vi "Config Sequence.vi"(8 "error in (no error)":errorcluster, 11 "STEPs":T1[](array[typedef])) -> (0 "error out":errorcluster, 3 "STEPs Out":T1[](array[typedef]))   [LabVIEW 2014, in "SeqLoop.lvlib"]
doc: "Configura las Mediciones."
uses:
  SeqLoop.lvlib
  TypeDefs/STEP.ctl
  TypeDefs/LogicParsedExpression.ctl
  Mimico Display/TypeDefs/Mimic Data.ctl
  Mimico Display/TypeDefs/BG Image.ctl
  Mimico Display/TypeDefs/mObject.ctl
  <vilib>/regexp/Match Regular Expression.xnode
  Mimico Display/Mimico Display.lvlib
panel:
  in  "Ver Seq":bool
  in  "Stop Seq":bool
  in  "Delete Seq":bool
  in  "Add Seq":bool
  in  "Secuencias":i32(listbox)=-1 caption="Secuencia"
  in  "Edit Seq":bool
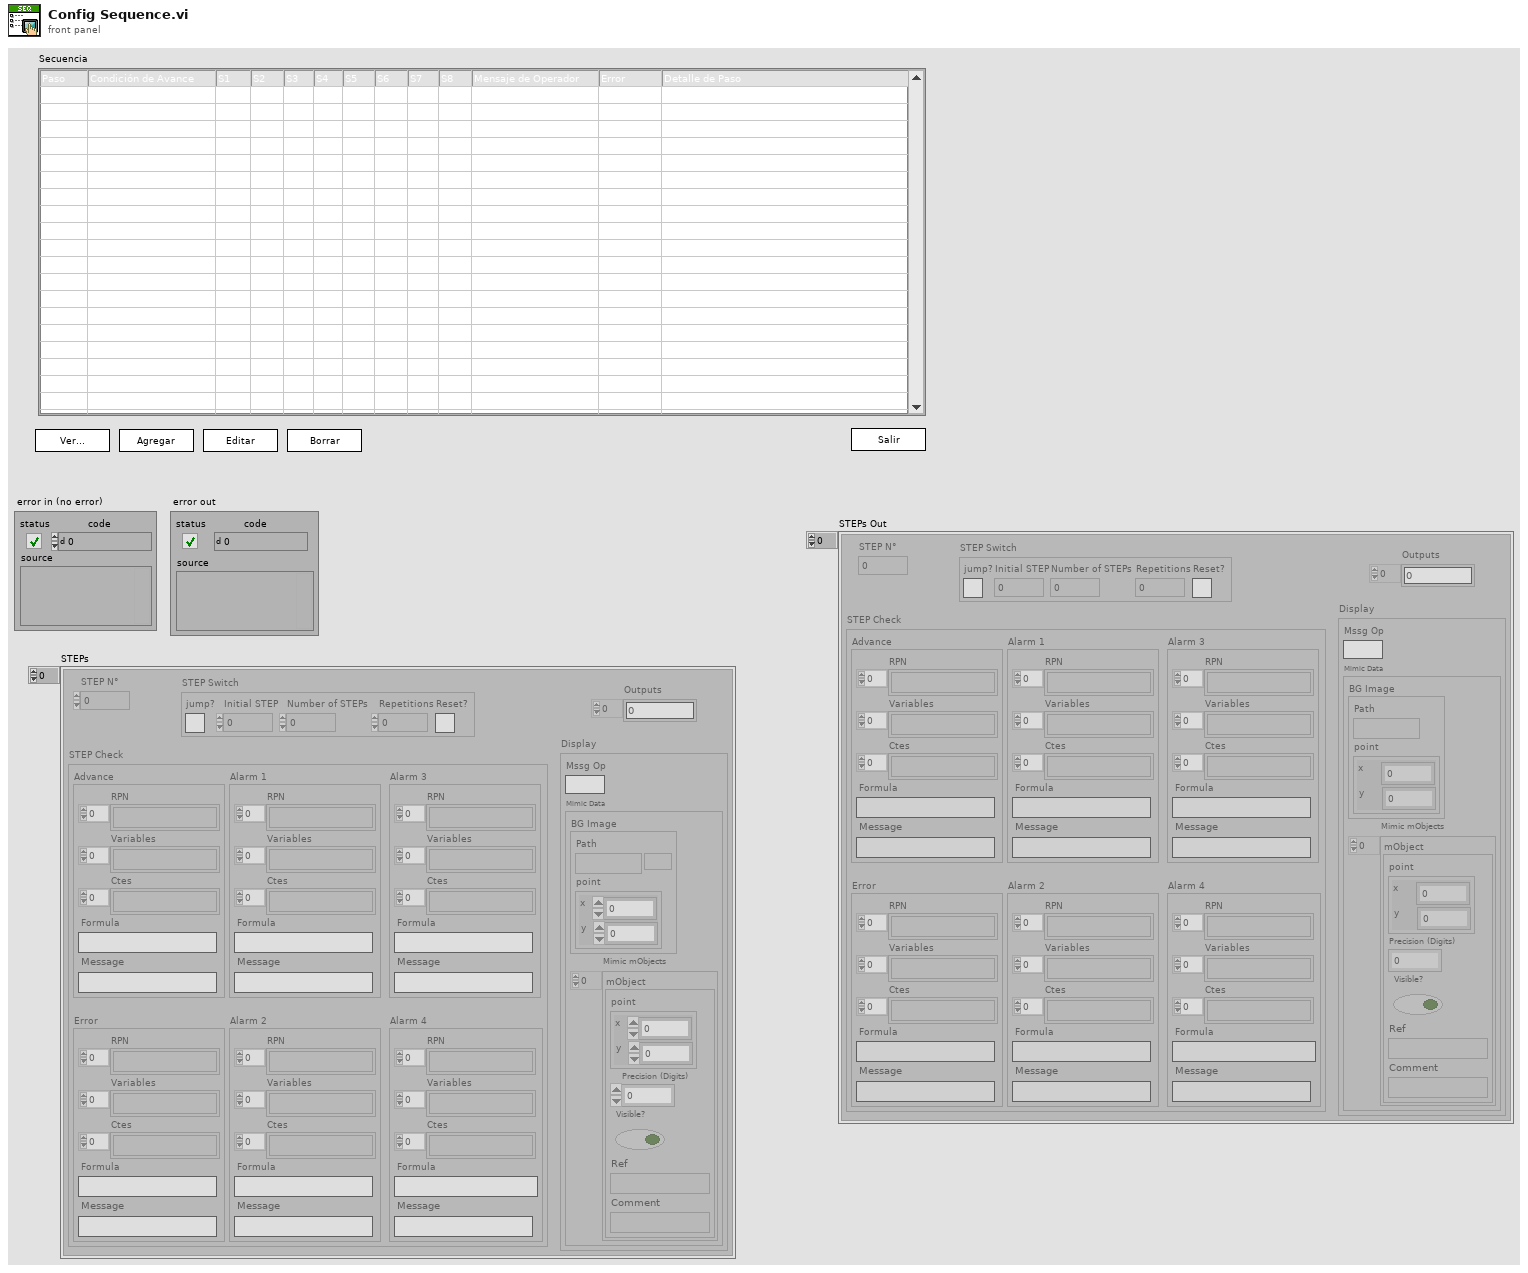
[diagram p1: front panel]
types:
  T1 = typedef "SeqLoop.lvlib/STEP.ctl" = cluster{"STEP N°":u32, "STEP Switch":cluster{"jump?":bool, "Initial STEP":u32, "Number of STEPs":u32, "Repetitions":u32, "Reset?":bool}, "Outputs":i32[], "STEP Check":cluster{"Advance":T2, "Error ":T2, "Alarm 1":T2, "Alarm 2":T2, "Alarm 3":T2, "Alarm 4":T2}, "Display":cluster{"Mssg Op":string, "Mimic Data":T3}}
  T2 = typedef "SeqLoop.lvlib/LogicParsedExpression.ctl" = cluster{"RPN ":string[], "Variables":string[], "Ctes":string[], "Formula":string, "Message":string}
  T3 = typedef "SeqLoop.lvlib/Mimico Display.lvlib/Mimic Data.ctl" = cluster{"BG Image":T4, "Mimic mObjects":T5[]}
  T4 = typedef "SeqLoop.lvlib/Mimico Display.lvlib/BG Image.ctl" = cluster{"Path":path, "point":cluster{"x":i16, "y":i16}}
  T5 = typedef "SeqLoop.lvlib/Mimico Display.lvlib/mObject.ctl" = cluster{"point":cluster{"x":i16, "y":i16}, "Precision (Digits)":i32, "Visible?":bool, "Ref":string, "Comment":string}
  T6 = enum8{"Enabled", "Disabled", "Disabled and Grayed Out"}
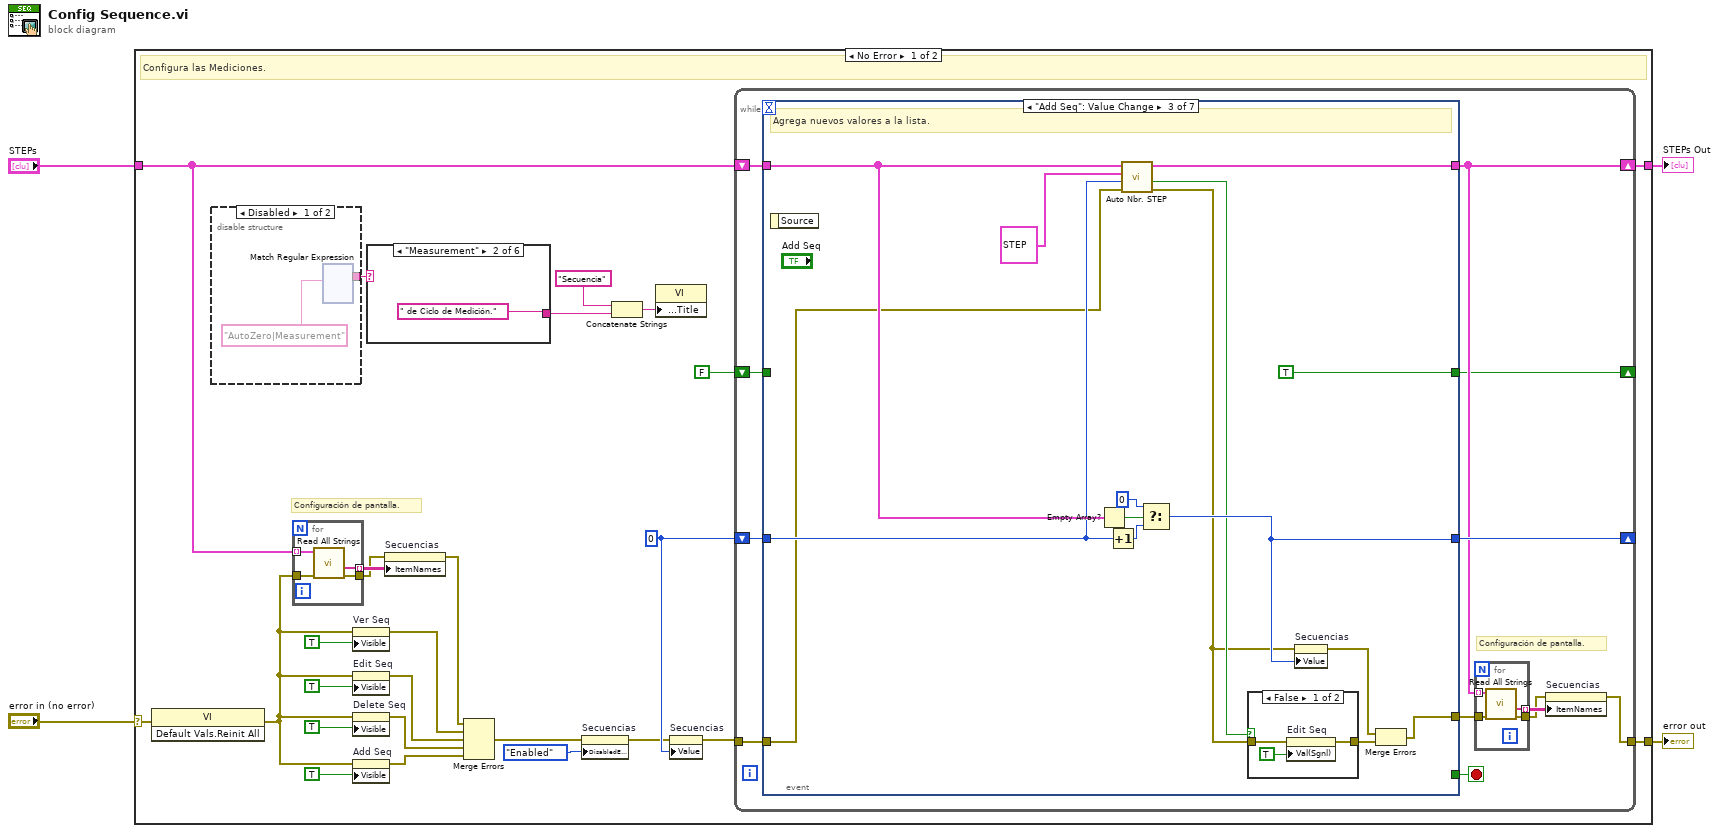
[diagram p0: block diagram]
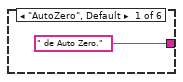
[diagram p3: hidden frame]
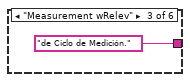
[diagram p4: hidden frame]
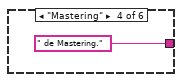
[diagram p5: hidden frame]
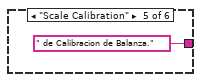
[diagram p6: hidden frame]
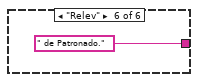
[diagram p7: hidden frame]
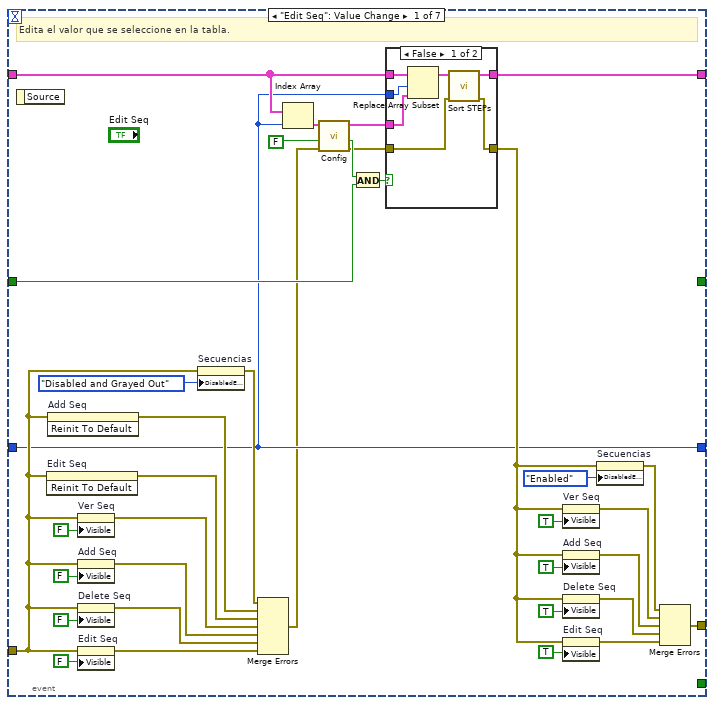
[diagram p8: hidden frame]
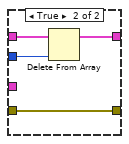
[diagram p9: hidden frame]
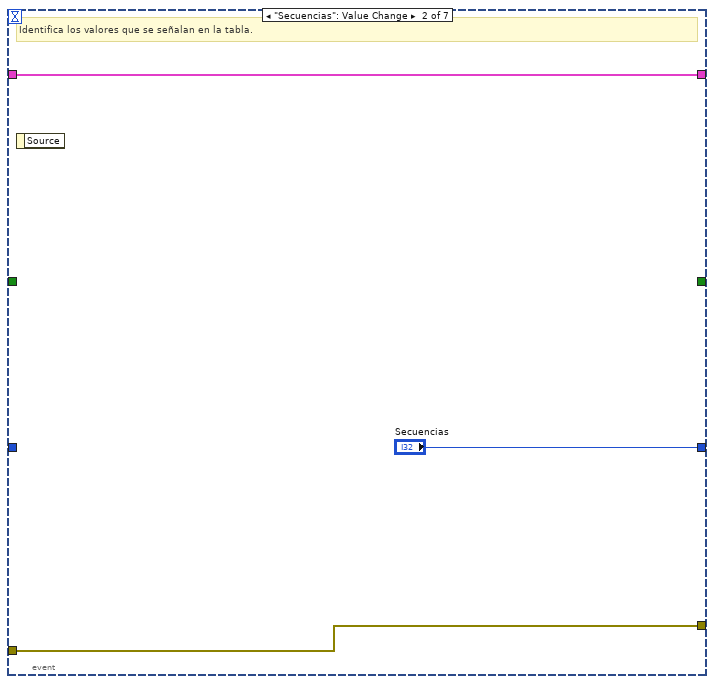
[diagram p10: hidden frame]
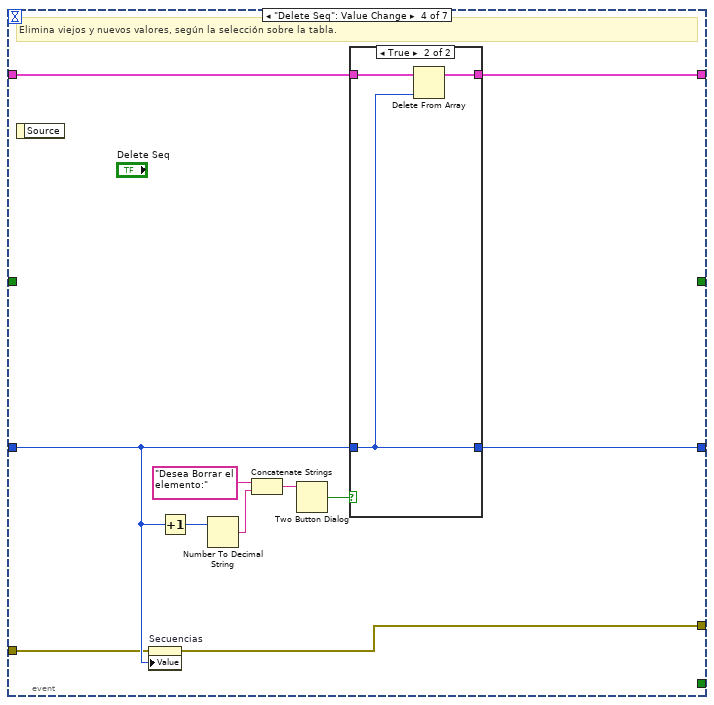
[diagram p12: hidden frame]
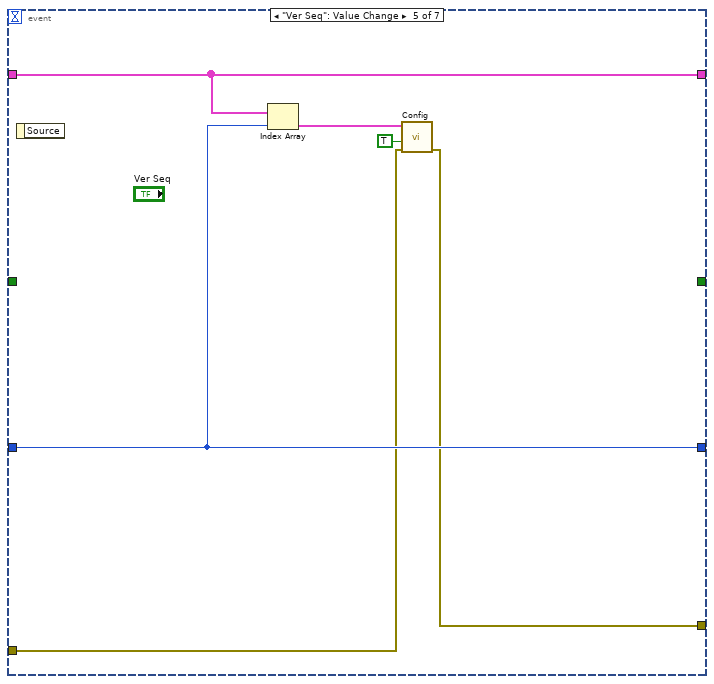
[diagram p14: hidden frame]
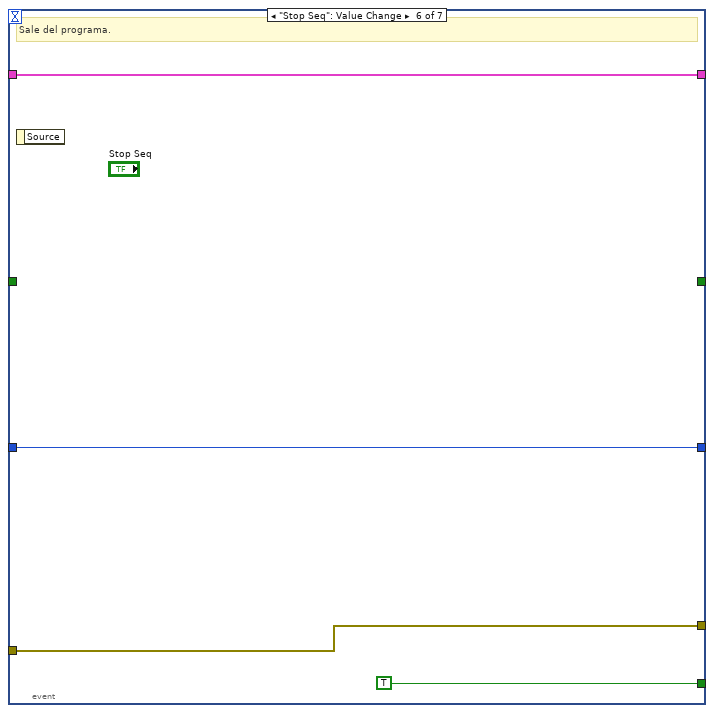
[diagram p15: hidden frame]
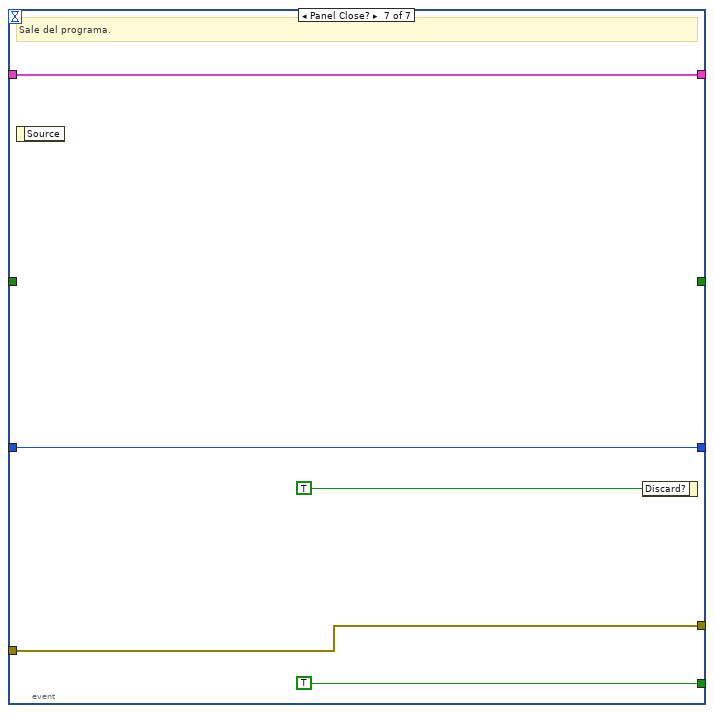
[diagram p16: hidden frame]
diagram:
  n1 = case shown="No Error" "error in (no error)" {
    selector: "error in (no error)" -> [w18 w273]
    tunnel: [w30 w273] -> w4
    tunnel: [w23 w274] -> w1
    tunnel: "STEPs" -> [w5 w274]
    frame No Error {
      w20 = 0 ("disabled index (col)")
      # "Configuración de pantalla."
      # "Configura las Mediciones."
      n2 = invoke class="VI" method="Default Vals.Reinit All"(error in=w18) -> (error out=w13:errorcluster)  [unwired: 2 in, 2 out]
      n3 = disable-structure shown="Disabled" {
        disable-tunnel: [w31 _] -> w9
        frame Disabled {
          n4 = xnode "Match Regular Expression"("regular expression"="AutoZero|Measurement") -> ("whole match"=w31:string)  [unwired: 5 in, 4 out]
        }
        frame Enabled {
        }
      }
      n5 = for {
        tunnel: w13 -> [w155]
        tunnel: [w156] -> w22 mode=indexing
        tunnel: [w154] -> w21
        tunnel: w5 -> [w153] mode=indexing
        n6 = call "Read All Strings.vi"("error in (no error)"=w155, "STEP in"=w153) -> ("error out"=w154:errorcluster, "All Strings"=w156:string[])  [unwired: 7 in, 1 out]
      }
      n7 = property on="Ver Seq" class="Bool"(error in=w13, "Visible"=TRUE) -> (error out=w12:errorcluster)  [unwired: 1 in, 1 out]
      n8 = property on="Edit Seq" class="Bool (strict)"(error in=w13, "Visible"=TRUE) -> (error out=w28:errorcluster)  [unwired: 1 in, 1 out]
      n9 = property on="Delete Seq" class="Bool"(error in=w13, "Visible"=TRUE) -> (error out=w26:errorcluster)  [unwired: 1 in, 1 out]
      n10 = property on="Add Seq" class="Bool (strict)"(error in=w13, "Visible"=TRUE) -> (error out=w24:errorcluster)  [unwired: 1 in, 1 out]
      n11 = case shown="\"Measurement\"" w9 {
        tunnel: [" de Auto Zero." ("Program Type") " de Ciclo de Medición." ("Program Type") "de Ciclo de Medición." ("Program Type") " de Mastering." ("Program Type") " de Calibracion de Balanza." ("Program Type") " de Patronado." ("Program Type")] -> w6
        frame "AutoZero", Default {
        }
        frame "Measurement" {
        }
        frame "Measurement wRelev" {
        }
        frame "Mastering" {
        }
        frame "Scale Calibration" {
        }
        frame "Relev" {
        }
      }
      n12 = property on="Secuencias" class="MCListbox (strict)"(error in=w21, "ItemNames"=w22) -> (error out=w11:errorcluster)  [unwired: 1 in, 1 out]
      n13 = Merge Errors(w11, w12, w28, w26, w24) -> (w17:errorcluster)
      n14 = property on="Secuencias" class="MCListbox (strict)"(error in=w17, "DisabledEnum"=T6."Enabled" ("Disabled")) -> (error out=w16:errorcluster)  [unwired: 1 in, 1 out]
      n15 = Concatenate Strings("Secuencia" ("Program Type"), w6) -> (w8:string)
      n16 = property class="VI"("Front Panel.Title"=w8) -> ()  [unwired: 2 in, 2 out]
      n17 = property on="Secuencias" class="MCListbox (strict)"(error in=w16, "Value"=w20) -> (error out=w15:errorcluster)  [unwired: 1 in, 1 out]
      n18 = while {
        shift-right: [w163] -> w23
        shift-left: w5 -> [w164]
        shift-right: [w165] -> _
        shift-left: w20 -> [w166]
        tunnel: w15 -> [w168]
        tunnel: [w159] -> w30
        shift-right: [w158] -> _
        shift-left: FALSE -> [w157]
        stop <- w167 stop-if-true
        # "Configuración de pantalla."
        n19 = event shown="[2] \"Add Seq\": Value Change" {
          selector: _ -> [_ _ _ _ _ _ _]
          dyn-events: _ -> [_ _ _ _ _ _ _]
          timeout: _ -> [_ _ _ _ _ _ _]
          tunnel: w164 -> [w179 w222 w232 w250 w263 w266 w272]
          tunnel: [w201 w222 w233 w249 w263 w266 w272] -> w163
          tunnel: [w178 "Secuencias" w227 w251 w262 w265 w271] -> w165
          tunnel: w166 -> [w178 _ w229 w244 w262 w265 w271]
          tunnel: w168 -> [w202 w220 w224 w243 w261 w267 w269]
          tunnel: [w184 w220 w235 w242 w260 w267 w269] -> w161
          tunnel: [_ _ _ _ _ TRUE ("Stop Med") TRUE ("Stop Med")] -> w167
          tunnel: [_ _ TRUE _ _ _ _] -> w158
          tunnel: w157 -> [w182 _ _ _ _ _ _]
          event "Edit Seq": Value Change {
            # "Edita el valor que se seleccione en la tabla."
            n20 = event-data() -> ()  [unwired: 1 in, 1 out]
            n21 = invoke on="Edit Seq" class="Bool (strict)" method="Reinit To Default"(error in=w202) -> (error out=w198:errorcluster)  [unwired: 2 in, 2 out]
            n22 = invoke on="Add Seq" class="Bool (strict)" method="Reinit To Default"(error in=w202) -> (error out=w197:errorcluster)  [unwired: 2 in, 2 out]
            n23 = property on="Ver Seq" class="Bool"(error in=w202, "Visible"=FALSE) -> (error out=w200:errorcluster)  [unwired: 1 in, 1 out]
            n24 = property on="Add Seq" class="Bool (strict)"(error in=w202, "Visible"=FALSE) -> (error out=w205:errorcluster)  [unwired: 1 in, 1 out]
            n25 = property on="Delete Seq" class="Bool"(error in=w202, "Visible"=FALSE) -> (error out=w199:errorcluster)  [unwired: 1 in, 1 out]
            n26 = property on="Edit Seq" class="Bool (strict)"(error in=w202, "Visible"=FALSE) -> (error out=w195:errorcluster)  [unwired: 1 in, 1 out]
            n27 = property on="Secuencias" class="MCListbox (strict)"(error in=w202, "DisabledEnum"=T6."Disabled and Grayed Out" ("Disabled")) -> (error out=w196:errorcluster)  [unwired: 1 in, 1 out]
            n28 = Merge Errors(w196, w197, w198, w200, w205, w199, w195) -> (w177:errorcluster)
            n29 = Index Array(array=w179, index=w178) -> (element=w176:T1)
            n30 = call "Config.vi"("error in (no error)"=w177, "Read only?"=FALSE ("View?"), "STEP in"=w176) -> ("error out"=w173:errorcluster, "Discard?"=w174:bool, "STEP out"=w175:T1)  [unwired: 6 in]
            n31 = And(x=w174, y=w182) -> (x .and. y?=w181:bool)
            n32 = case shown="False" w181 {
              tunnel: w179 -> [w215 w218]
              tunnel: w178 -> [w214 w216]
              tunnel: w175 -> [w213 _]
              tunnel: [w211 w217] -> w201
              tunnel: w173 -> [w210 w219]
              tunnel: [w209 w219] -> w185
              frame False {
                n33 = Replace Array Subset(array=w215, new element=w213, index=w214) -> (w212:T1[])
                n34 = call "Sort STEPs.vi"("error in (no error)"=w210, "STEPs In"=w212) -> ("error out"=w209:errorcluster, "STEPs Out"=w211:T1[])  [unwired: 8 in]
              }
              frame True {
                n35 = Delete From Array(array=w218, index=w216) -> (array with subset deleted=w217:T1[])  [unwired: 1 in, 1 out]
              }
            }
            n36 = property on="Ver Seq" class="Bool"(error in=w185, "Visible"=TRUE) -> (error out=w192:errorcluster)  [unwired: 1 in, 1 out]
            n37 = property on="Add Seq" class="Bool (strict)"(error in=w185, "Visible"=TRUE) -> (error out=w189:errorcluster)  [unwired: 1 in, 1 out]
            n38 = property on="Delete Seq" class="Bool"(error in=w185, "Visible"=TRUE) -> (error out=w193:errorcluster)  [unwired: 1 in, 1 out]
            n39 = property on="Edit Seq" class="Bool (strict)"(error in=w185, "Visible"=TRUE) -> (error out=w194:errorcluster)  [unwired: 1 in, 1 out]
            n40 = property on="Secuencias" class="MCListbox (strict)"(error in=w185, "DisabledEnum"=T6."Enabled" ("Disabled")) -> (error out=w183:errorcluster)  [unwired: 1 in, 1 out]
            n41 = Merge Errors(w183, w192, w189, w193, w194) -> (w184:errorcluster)
          }
          event "Secuencias": Value Change {
            # "Identifica los valores que se señalan en la tabla."
            n42 = event-data() -> ()  [unwired: 1 in, 1 out]
          }
          event "Add Seq": Value Change {
            # "Agrega nuevos valores a la lista."
            n43 = event-data() -> ()  [unwired: 1 in, 1 out]
            n44 = Empty Array?(array=w232) -> (empty?=w231:bool)
            n45 = Increment(x=w229) -> (x+1=w228:i32)
            n46 = call "Auto Nbr. STEP.vi"("error in (no error)"=w224, "index (col)"=w229, "STEP in"=T1 {"STEP N°"=0, "STEP Switch"={"jump?"=FALSE, "Initial STEP"=0, "Number of STEPs"=0, "Repetitions"=0, "Reset?"=FALSE}, "Outputs"=[], "STEP Check"={"Advance"={"RPN "=[], "Variables"=[], "Ctes"=[], "Formula"="", "Message"=""}, "Error "={"RPN "=[], "Variables"=[], "Ctes"=[], "Formula"="", "Message"=""}, "Alarm 1"={"RPN "=[], "Variables"=[], "Ctes"=[], "Formula"="", "Message"=""}, "Alarm 2"={"RPN "=[], "Variables"=[], "Ctes"=[], "Formula"="", "Message"=""}, "Alarm 3"={"RPN "=[], "Variables"=[], "Ctes"=[], "Formula"="", "Message"=""}, "Alarm 4"={"RPN "=[], "Variables"=[], "Ctes"=[], "Formula"="", "Message"=""}}, "Display"={"Mssg Op"="", "Mimic Data"={"BG Image"={"Path"=path "", "point"={"x"=0, "y"=0}}, "Mimic mObjects"=[]}}} ("STEP"), "STEPs In"=w232) -> ("error out"=w225:errorcluster, "Discarded?"=w226:bool, "STEPs Out"=w233:T1[])  [unwired: 5 in]
            n47 = Select(t=0 ("disabled index (col)"), s=w231, f=w228) -> (s? t:f=w227:i32)
            n48 = case shown="False" w226 {
              tunnel: [w240 w241] -> w237
              tunnel: w225 -> [w239 w241]
              frame False {
                n49 = property on="Edit Seq" class="Bool (strict)"(error in=w239, "Val(Sgnl)"=TRUE ("Value (Signaling)")) -> (error out=w240:errorcluster)  [unwired: 1 in, 1 out]
              }
              frame True {
              }
            }
            n50 = property on="Secuencias" class="MCListbox (strict)"(error in=w225, "Value"=w227) -> (error out=w236:errorcluster)  [unwired: 1 in, 1 out]
            n51 = Merge Errors(w236, w237) -> (w235:errorcluster)
          }
          event "Delete Seq": Value Change {
            # "Elimina viejos y nuevos valores, según la selección sobre la tabla."
            n52 = event-data() -> ()  [unwired: 1 in, 1 out]
            n53 = property on="Secuencias" class="MCListbox (strict)"(error in=w243, "Value"=w244) -> (error out=w242:errorcluster)  [unwired: 1 in, 1 out]
            n54 = Increment(x=w244) -> (x+1=w245:i32)
            n55 = Number To Decimal String(number=w245) -> (decimal integer string=w247:string)  [unwired: 1 in]
            n56 = Concatenate Strings("Desea Borrar el elemento:" ("message"), w247) -> (w246:string)
            n57 = Two Button Dialog(message=w246) -> (T button?=w252:bool)  [unwired: 2 in]
            n58 = case shown="True" w252 {
              tunnel: w250 -> [w253 w257]
              tunnel: [w254 w255] -> w251
              tunnel: w244 -> [w254 w255]
              tunnel: [w253 w256] -> w249
              frame False {
              }
              frame True {
                n59 = Delete From Array(array=w257, index=w255) -> (array with subset deleted=w256:T1[])  [unwired: 1 in, 1 out]
              }
            }
          }
          event "Ver Seq": Value Change {
            n60 = event-data() -> ()  [unwired: 1 in, 1 out]
            n61 = Index Array(array=w263, index=w262) -> (element=w258:T1)
            n62 = call "Config.vi"("error in (no error)"=w261, "Read only?"=TRUE ("View?"), "STEP in"=w258) -> ("error out"=w260:errorcluster)  [unwired: 6 in, 2 out]
          }
          event "Stop Seq": Value Change {
            # "Sale del programa."
            n63 = event-data() -> ()  [unwired: 1 in, 1 out]
          }
          event Panel Close? {
            # "Sale del programa."
            n64 = event-data() -> ()  [unwired: 1 in, 1 out]
            n65 = event-data("Discard?"=TRUE) -> ()  [unwired: 1 in, 1 out]
          }
        }
        n66 = for {
          tunnel: w163 -> [w172] mode=indexing
          tunnel: w161 -> [w170]
          tunnel: [w171] -> w162 mode=indexing
          tunnel: [w169] -> w160
          n67 = call "Read All Strings.vi"("error in (no error)"=w170, "STEP in"=w172) -> ("error out"=w169:errorcluster, "All Strings"=w171:string[])  [unwired: 7 in, 1 out]
        }
        n68 = property on="Secuencias" class="MCListbox (strict)"(error in=w160, "ItemNames"=w162) -> (error out=w159:errorcluster)  [unwired: 1 in, 1 out]
      }
    }
    frame Error {
    }
  }
  "error out" <- w4
  "STEPs Out" <- w1
